vi "Request Channel Names.vi"(7 "Source ID":u32, 10 "Group":refnum<class "Group.lvclass">, 11 "Discovery":refnum<class "NodeDiscovery.lvclass">) -> ()   [LabVIEW 2020, in "Vecto.lvlib" / "RemoteDataService.lvclass"]
uses:
  RemoteDataService.lvclass
  RemoteDataService.lvclass/RemoteDataService.ctl
  Request Channel Names Async.vi
  Group/Group.lvclass
  NodeDiscovery/NodeDiscovery.lvclass
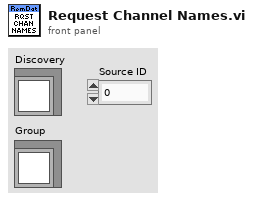
[diagram p1: front panel]
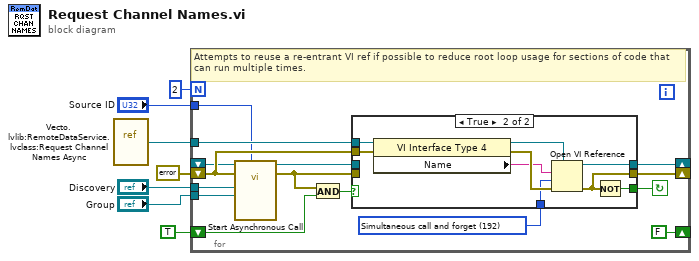
[diagram p0: block diagram]
diagram:
  n1 = vi-ref "Vecto.lvlib:RemoteDataService.lvclass:Request Channel Names Async.vi"() -> (w7:refnum<vi>)
  n2 = for {
    N: 2 -> [_]
    tunnel: w7 -> [w21]
    shift-right: [w20] -> _
    shift-left: _ -> [w19]
    shift-right: [w17] -> _
    shift-left: errorcluster {"status"=FALSE, "code"=0, "source"=""} ("error constant") -> [w22]
    shift-right: [FALSE] -> _
    shift-left: TRUE -> [w14]
    tunnel: "Source ID" -> [w10]
    tunnel: "Discovery" -> [w9]
    tunnel: "Group" -> [w8]
    stop <- w13 continue-if-true
    w11 = 192 items=["Record modifications"=1, "Open templates for editing"=2, "Prompt user to save"=4, "Prepare for reentrant run"=8, "Prompt to find missing subVIs"=16, "Hide loading dialog box"=32, "Enable simultaneous calls"=64, "Prepare to call and forget"=128, "Simultaneous call and forget"=192, "Prepare to call and collect"=256, "Simultaneous call and collect"=320]
    # "Attempts to reuse a re-entrant VI ref if possible to reduce root loop usage for sections of code that can run multiple times."
    n3 = call-by-ref "Start Asynchronous Call"(reference=w19, error in=w22, "Source ID"=w10, "Group"=w8, "Discovery"=w9) -> (reference out=w18:refnum<vi>, error out=w16:errorcluster)  [unwired: 9 in]
    n4 = And(x=w16, y=w14) -> (x .and. y?=w15:bool)
    n5 = case shown="True" w15 {
      tunnel: w21 -> [_ w32]
      tunnel: w11 -> [_ w30]
      tunnel: [w24 w28] -> w20
      tunnel: w18 -> [w24 _]
      tunnel: [w23 w26] -> w17
      tunnel: w16 -> [w23 _]
      tunnel: w22 -> [_ w27]
      tunnel: [_ w25] -> w13
      frame False {
      }
      frame True {
        n6 = property class="VI Interface Type 4"(reference=w32, error in=w27) -> (reference out=w29:refnum<vi>, error out=w33:errorcluster, "Name"=w31:string)
        n7 = Open VI Reference(type specifier VI Refnum (for type only)=w29, vi path=w31, options=w30, error in (no error)=w33) -> (vi reference=w28:refnum<vi>, error out=w26:errorcluster)  [unwired: 2 in]
        n8 = Not(x=w26) -> (.not. x?=w25:bool)
      }
    }
  }
